vi "Read classes path.vi"(8 "error in (no error)":errorcluster, 11 "Repository in":refnum<class "Repository.lvclass">) -> (0 "error out":errorcluster, 2 "classes path":path, 3 "Repository out":refnum<class "Repository.lvclass">)   [LabVIEW 2013]
uses:
  Repository.lvclass
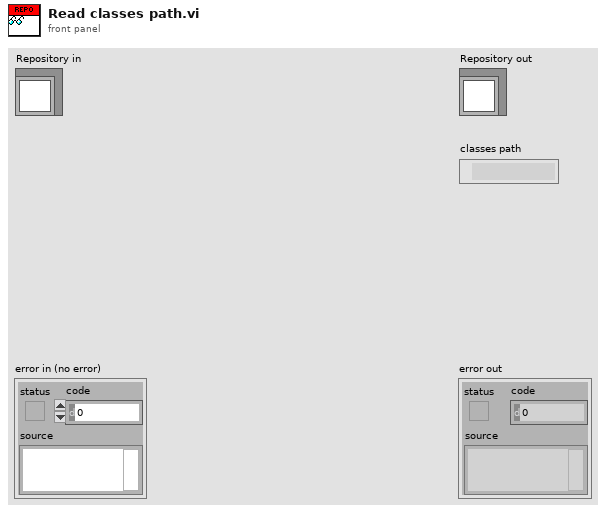
[diagram p1: front panel]
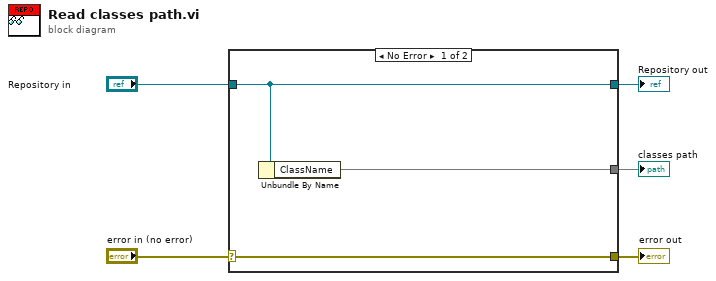
[diagram p0: block diagram]
diagram:
  n1 = case shown="No Error" "error in (no error)" {
    selector: "error in (no error)" -> [w8 w9]
    tunnel: [w8 w9] -> w4
    tunnel: [w7 w10] -> w2
    tunnel: "Repository in" -> [w7 w10]
    tunnel: [w6 _] -> w1
    frame No Error {
      n2 = Unbundle By Name(w7) -> ("ClassName"=w6)
    }
    frame Error {
    }
  }
  "error out" <- w4
  "Repository out" <- w2
  "classes path" <- w1
